vi "Acquire UDP Data.vi"(6 "Infm Alive Counter":u16, 8 "error in":errorcluster, 11 "connection UDP in":refnum<k16>) -> (0 "error out":errorcluster, 1 "data out":string, 2 "Data Valid ?":bool, 3 "connection ID out":refnum<k16>, 4 "Infm Alive Counter out":u16)   [LabVIEW 2016, in "Acquisition.lvlib"]
doc: "Generates sample waveforms according to the signal type in the HW Config input.\n_____\nBased on DQMH Project Template 6.1.0.94."
uses:
  Acquisition.lvlib
  Signal Type--enum.ctl
  CML UI/CML UI.lvlib
panel:
  out "data out 2":string
  in  "Signal Type":T1
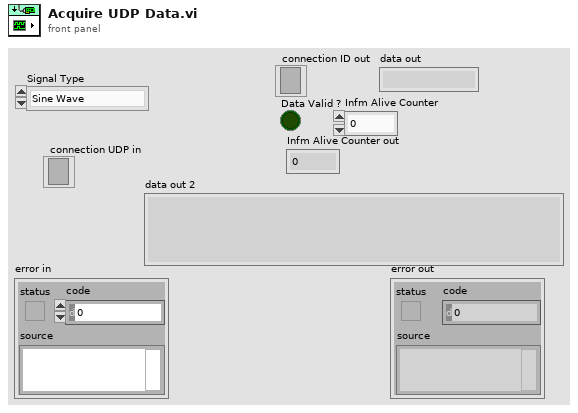
[diagram p1: front panel]
types:
  T1 = typedef "Acquisition.lvlib/Signal Type--enum.ctl" = enum16{"Sine Wave", "Square with Noise"}
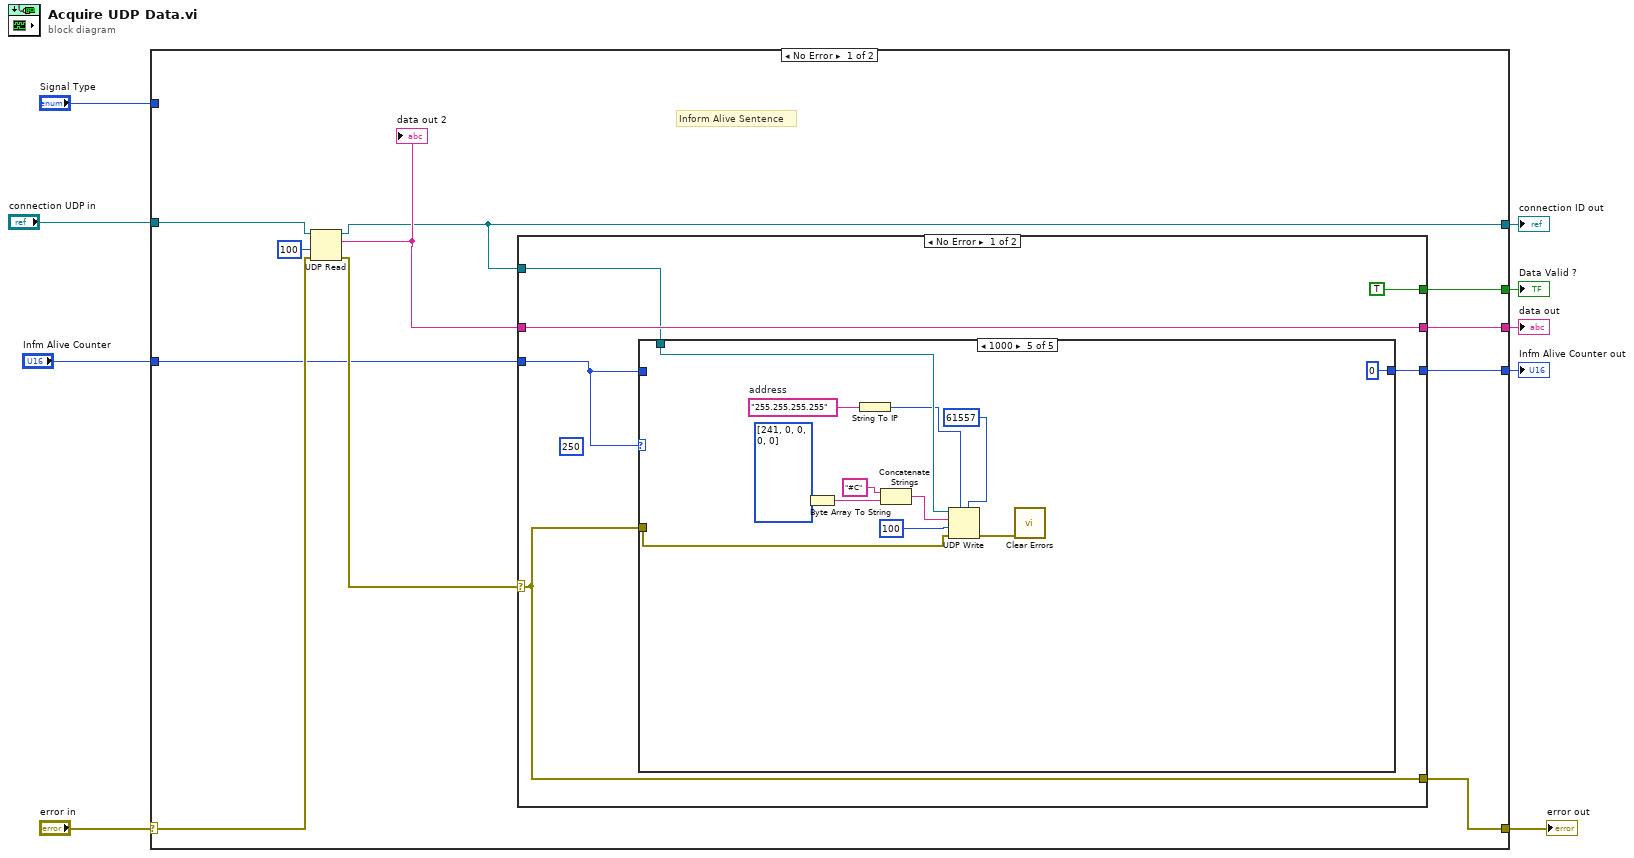
[diagram p0: block diagram]
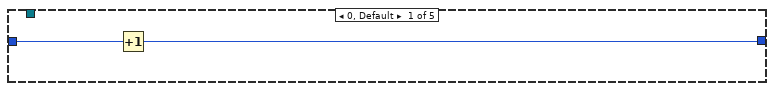
[diagram p2: hidden frame]
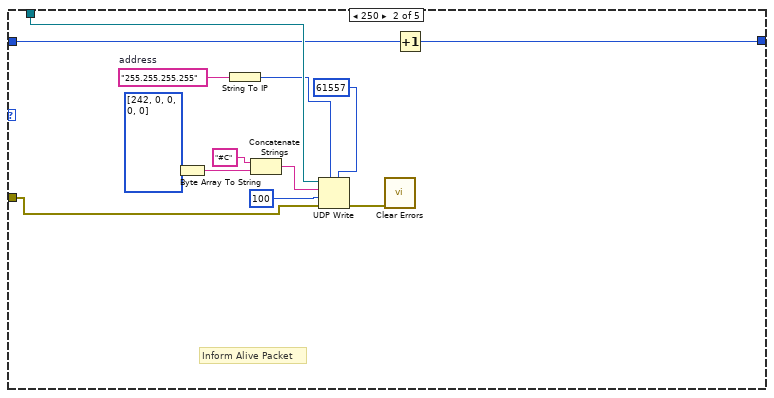
[diagram p3: hidden frame]
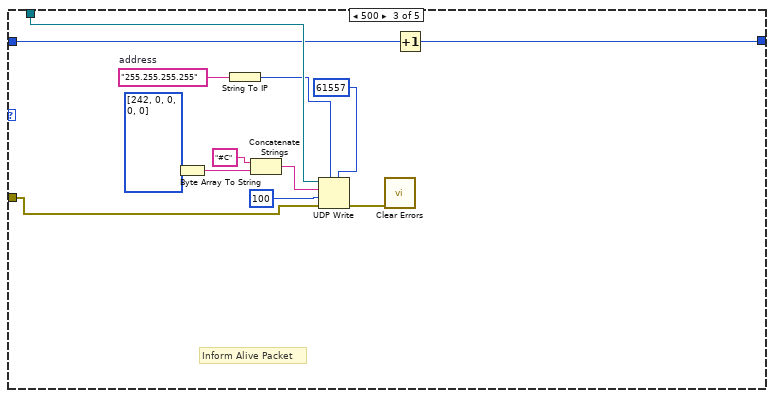
[diagram p4: hidden frame]
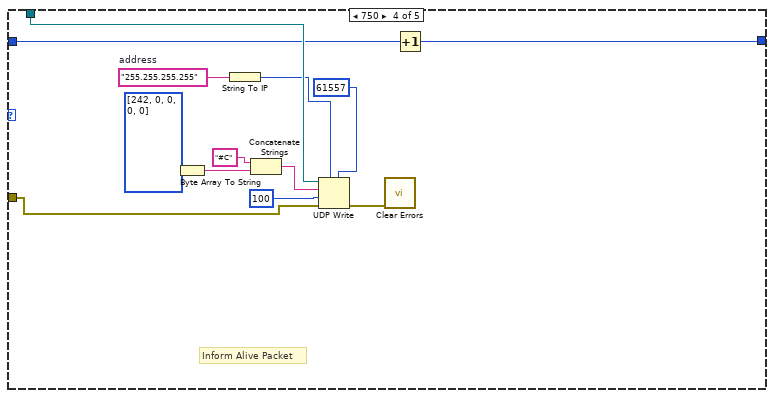
[diagram p5: hidden frame]
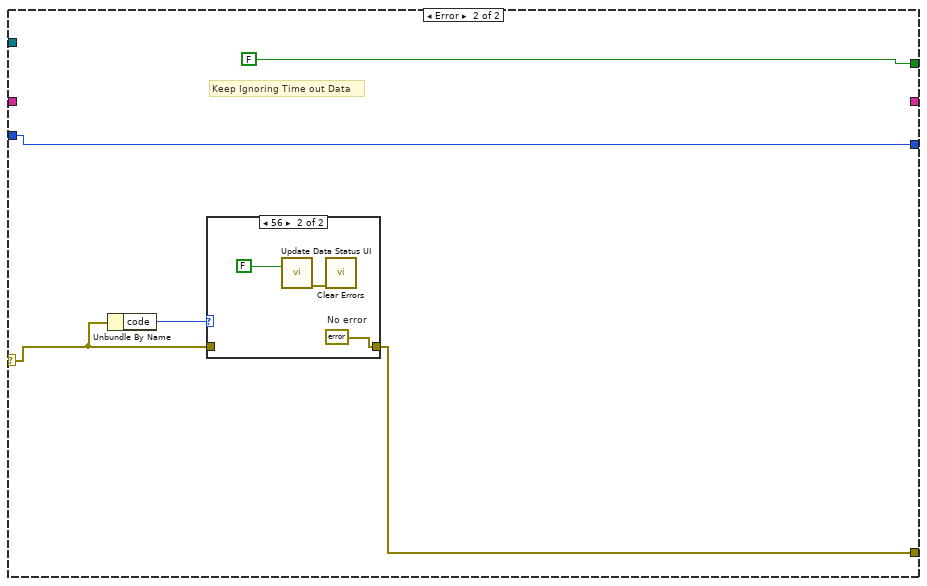
[diagram p6: hidden frame]
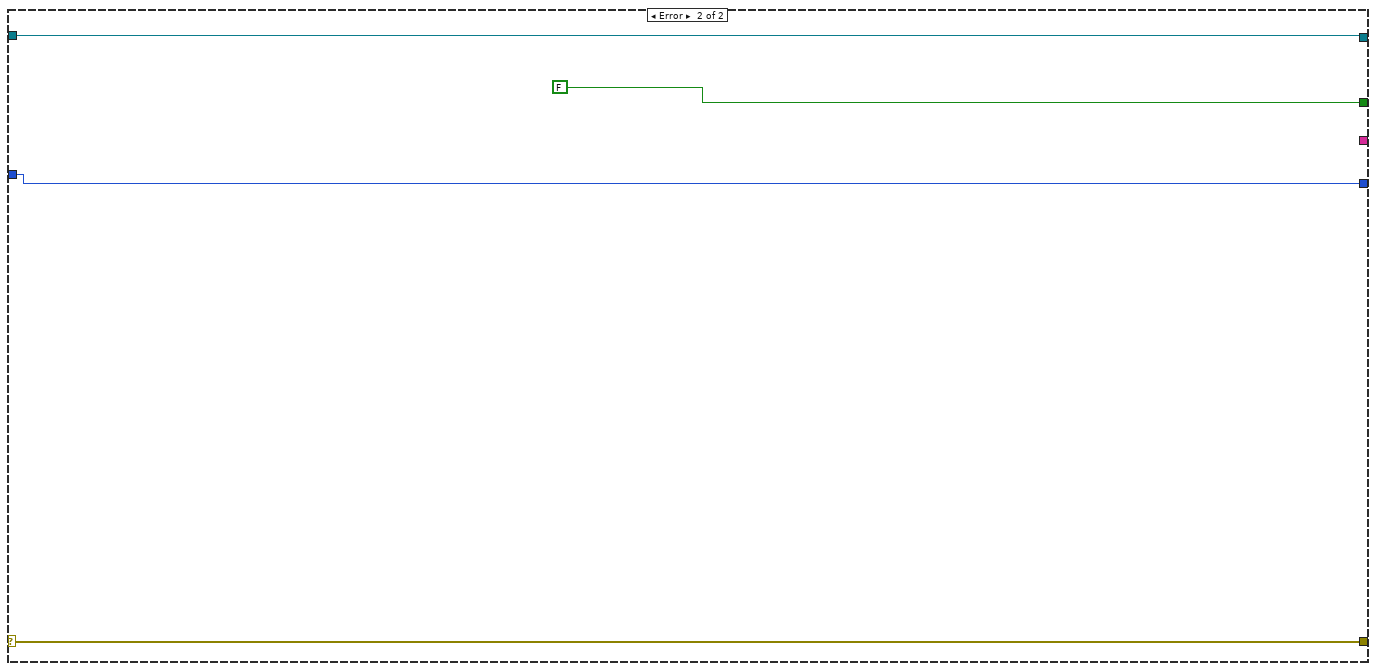
[diagram p8: hidden frame]
diagram:
  n1 = case shown="No Error" "error in" {
    selector: "error in" -> [w18 w92]
    tunnel: [w13 w92] -> w8
    tunnel: "Signal Type" -> [_ _]
    tunnel: "connection UDP in" -> [w19 w91]
    tunnel: [w10 w91] -> w5
    tunnel: [w15 _] -> w3
    tunnel: [w14 FALSE] -> w4
    tunnel: "Infm Alive Counter" -> [w12 w89]
    tunnel: [w11 w89] -> w1
    frame No Error {
      # "Inform Alive Sentence"
      n2 = UDP Read(connection ID=w19, timeout ms (25000)=100, 8:w18) -> (data out=w16:string, error out=w17:errorcluster, 3:w10:refnum<k16>)  [unwired: 3 out]
      "data out 2" <- w16
      n3 = case shown="No Error" w17 {
        selector: w17 -> [w22 w82]
        tunnel: w16 -> [w26 _]
        tunnel: [w26 _] -> w15
        tunnel: [TRUE FALSE] -> w14
        tunnel: [w22 w81] -> w13
        tunnel: w12 -> [w21 w80]
        tunnel: [w24 w80] -> w11
        tunnel: w10 -> [w23 _]
        frame No Error {
          (unwired) u16 250 ("y")
          n4 = case shown="1000" w21 {
            tunnel: [w27 w30 w43 w56 u16 0] -> w24
            tunnel: w21 -> [w28 w31 w44 w57 _]
            tunnel: w23 -> [_ w35 w48 w61 w73]
            tunnel: w22 -> [_ w36 w49 w62 w74]
            frame 0, Default {
              n5 = Increment(x=w28) -> (x+1=w27:u16)
            }
            frame 250 {
              w33 = "255.255.255.255"  # address
              # "Inform Alive Packet"
              n6 = Byte Array To String(unsigned byte array=u8[] [242, 0, 0, 0, 0]) -> (string=w40:string)
              n7 = String To IP(1:w33) -> (0:w32:u32)
              n8 = Concatenate Strings("#C", w40) -> (w37:string)
              n9 = UDP Write(address=w32, port or service name=u16 61557 ("remote port"), connection ID=w35, data in=w37, 8:w36, 9:100 ("timeout ms (25000)")) -> (error out=w29:errorcluster)  [unwired: 1 out]
              n10 = call <vilib>:"Clear Errors.vi"("error in (no error)"=w29) -> ()  [unwired: 5 in, 2 out]
              n11 = Increment(x=w31) -> (x+1=w30:u16)
            }
            frame 500 {
              w46 = "255.255.255.255"  # address
              # "Inform Alive Packet"
              n12 = Byte Array To String(unsigned byte array=u8[] [242, 0, 0, 0, 0]) -> (string=w53:string)
              n13 = String To IP(1:w46) -> (0:w45:u32)
              n14 = Concatenate Strings("#C", w53) -> (w50:string)
              n15 = UDP Write(address=w45, port or service name=u16 61557 ("remote port"), connection ID=w48, data in=w50, 8:w49, 9:100 ("timeout ms (25000)")) -> (error out=w42:errorcluster)  [unwired: 1 out]
              n16 = call <vilib>:"Clear Errors.vi"("error in (no error)"=w42) -> ()  [unwired: 5 in, 2 out]
              n17 = Increment(x=w44) -> (x+1=w43:u16)
            }
            frame 750 {
              w59 = "255.255.255.255"  # address
              # "Inform Alive Packet"
              n18 = Byte Array To String(unsigned byte array=u8[] [242, 0, 0, 0, 0]) -> (string=w66:string)
              n19 = String To IP(1:w59) -> (0:w58:u32)
              n20 = Concatenate Strings("#C", w66) -> (w63:string)
              n21 = UDP Write(address=w58, port or service name=u16 61557 ("remote port"), connection ID=w61, data in=w63, 8:w62, 9:100 ("timeout ms (25000)")) -> (error out=w55:errorcluster)  [unwired: 1 out]
              n22 = call <vilib>:"Clear Errors.vi"("error in (no error)"=w55) -> ()  [unwired: 5 in, 2 out]
              n23 = Increment(x=w57) -> (x+1=w56:u16)
            }
            frame 1000 {
              w71 = "255.255.255.255"  # address
              n24 = Byte Array To String(unsigned byte array=u8[] [241, 0, 0, 0, 0]) -> (string=w78:string)
              n25 = String To IP(1:w71) -> (0:w70:u32)
              n26 = Concatenate Strings("#C", w78) -> (w75:string)
              n27 = UDP Write(address=w70, port or service name=u16 61557 ("remote port"), connection ID=w73, data in=w75, 8:w74, 9:100 ("timeout ms (25000)")) -> (error out=w69:errorcluster)  [unwired: 1 out]
              n28 = call <vilib>:"Clear Errors.vi"("error in (no error)"=w69) -> ()  [unwired: 5 in, 2 out]
            }
          }
        }
        frame Error {
          # "Keep Ignoring Time out Data"
          n29 = Unbundle By Name(w82) -> ("code"=w83:i32)
          n30 = case shown="56" w83 {
            tunnel: w82 -> [w85 _]
            tunnel: [w85 w88] -> w81
            frame Default {
            }
            frame 56 {
              w88 = errorcluster {"status"=FALSE, "code"=0, "source"=""}  # No error
              n31 = call "Update Data Status UI.vi"("status"=FALSE) -> ("error out"=w86:errorcluster)  [unwired: 10 in]
              n32 = call <vilib>:"Clear Errors.vi"("error in (no error)"=w86) -> ()  [unwired: 5 in, 2 out]
            }
          }
        }
      }
    }
    frame Error {
    }
  }
  "error out" <- w8
  "connection ID out" <- w5
  "Data Valid ?" <- w4
  "data out" <- w3
  "Infm Alive Counter out" <- w1
